vi "wholeBrainImagerSetLasers.vi"() -> ()   [LabVIEW 2017]
uses:
  globalUtilities.vi
panel:
  out "slider position":i32
  # "SET THE LASERS TO THE POWERS \nNEEDED FOR THE WHOLE BRAIN IMAGER"
  # "Additionally, sets also the shutter/slider\nto the right position."
  # "should be 2"
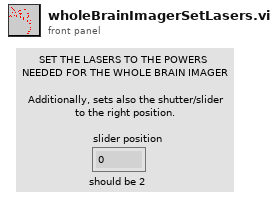
[diagram p1: front panel]
types:
  T1 = cluster{"laserWavelength (nm)":dbl, "laserPower (mW)":dbl, "sliderPosition":u16}[]
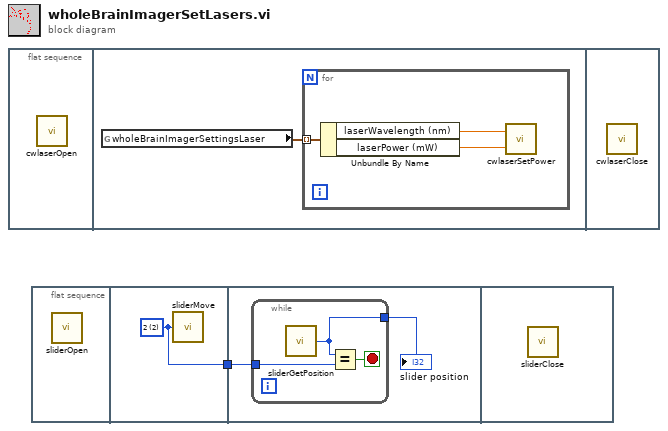
[diagram p0: block diagram]
diagram:
  n1 = flat-sequence {
    frame #0 {
      n2 = call "cwlaserOpen.vi"() -> ()  [unwired: 4 in]
    }
    frame #1 {
      n3 = global read "globalUtilities.vi" "wholeBrainImagerSettingsLaser"() -> (w2:T1)
      n4 = for {
        tunnel: w2 -> [w5] mode=indexing
        n5 = Unbundle By Name(w5) -> ("laserWavelength (nm)"=w4:dbl, "laserPower (mW)"=w3:dbl)
        n6 = call "cwlaserSetPower.vi"("power (mW)"=w3, "wavelength"=w4) -> ()  [unwired: 1 out]
      }
    }
    frame #2 {
      n7 = call "cwlaserClose.vi"() -> ()  [unwired: 3 in]
    }
  }
  n8 = flat-sequence {
    tunnel: [w6] -> w1
    tunnel: w1 -> [w8]
    frame #0 {
      n9 = call "sliderOpen.vi"() -> ()  [unwired: 1 in, 2 out]
    }
    frame #1 {
      w6 = u16 2 items=["0", "1", "2", "3"] ("position")
      n10 = call "sliderMove.vi"("position"=w6) -> ()  [unwired: 1 out]
    }
    frame #2 {
      n11 = while {
        tunnel: [w10] -> w7
        tunnel: w8 -> [w9]
        stop <- w11 stop-if-true
        n12 = call "sliderGetPosition.vi"() -> ("position"=w10:i32)  [unwired: 1 in]
        n13 = Equal?(x=w10, y=w9) -> (x = y?=w11:bool)
      }
      "slider position" <- w7
    }
    frame #3 {
      n14 = call "sliderClose.vi"() -> ()  [unwired: 2 in, 1 out]
    }
  }
